vi "XVC_SERVER_UDP.vi"() -> ()   [LabVIEW 2017]
panel:
  out "error out":errorcluster
  in  "data out 5":string="shift:\u0005\u0000\u0000\u0000ÿ\u0000"
  out "received string 2":string
  in  "address":string="192.168.10.35"
  out "received string":string
  out "data out 3":string
  in  "data out 4":string="shift:\u0005\u0000\u0000\u0000ÿ\u0000"
  out "data out 2":string
  out "x != 0?":bool
  in  "Client Closed":string="The client VI closed the connection."
  in  "Stop":bool
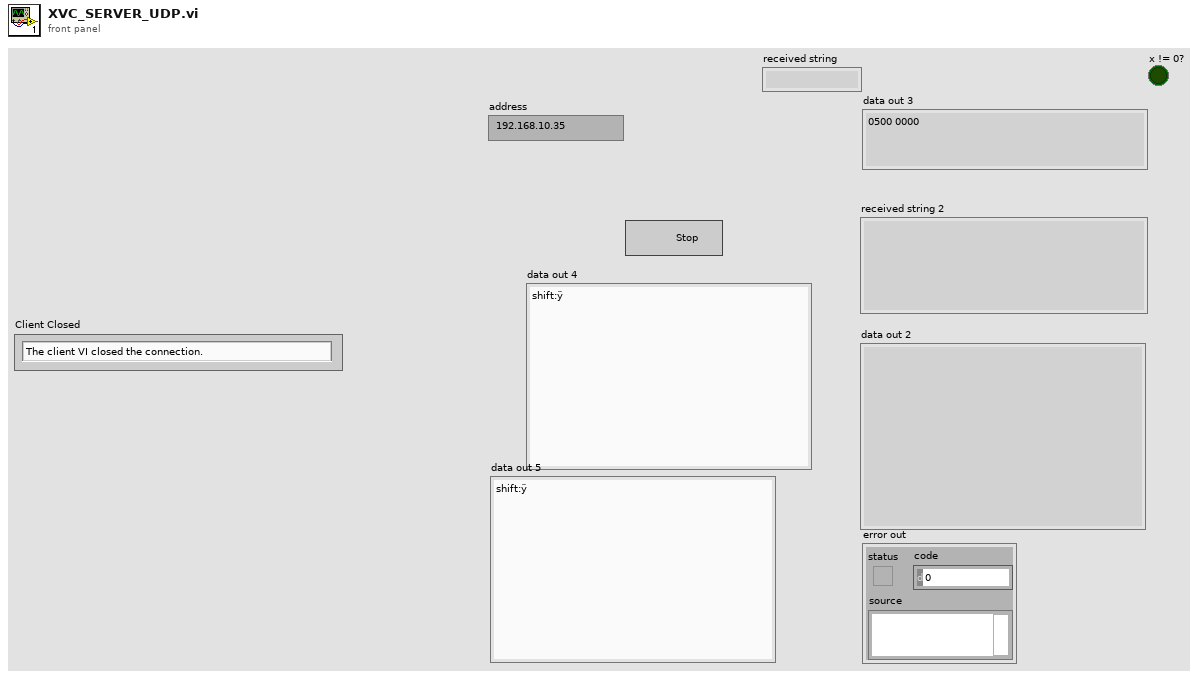
[diagram p1: front panel]
types:
  T1 = enum16{"Standard", "Buffered", "CRLF", "Immediate"}
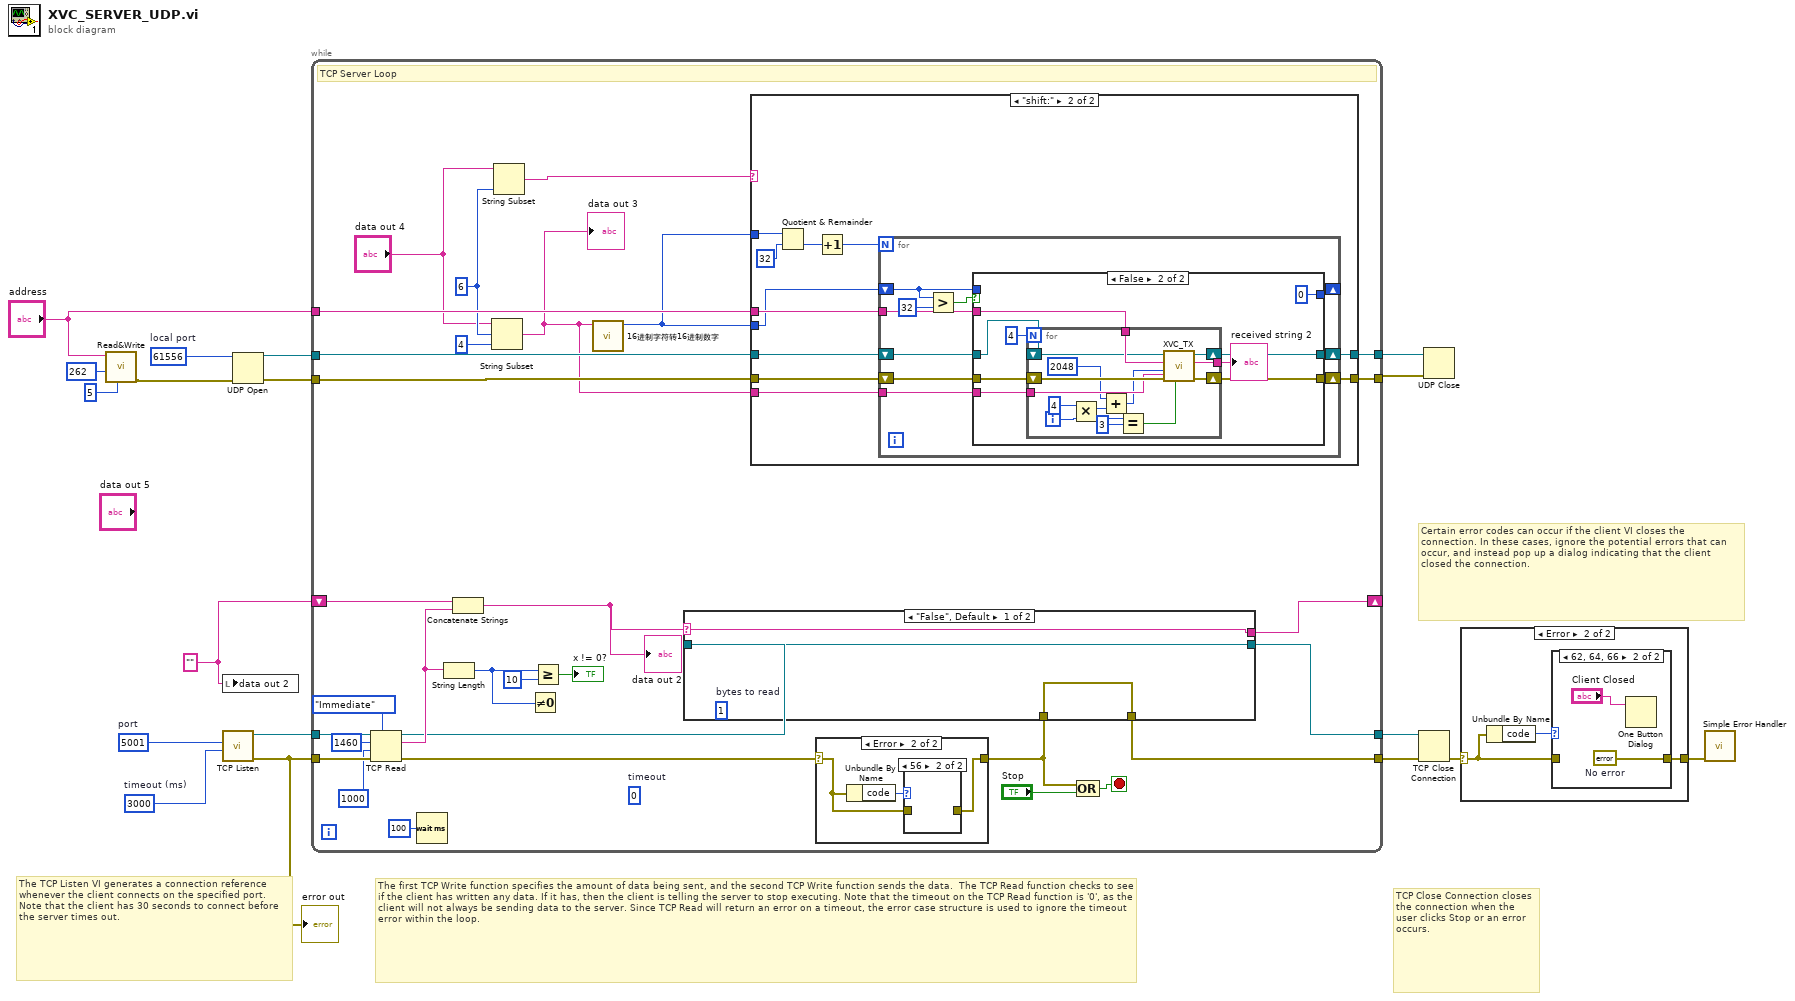
[diagram p0: block diagram]
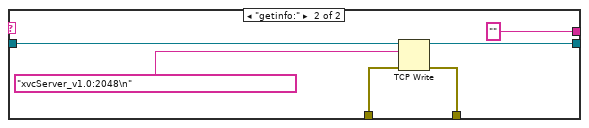
[diagram p4: hidden frame]
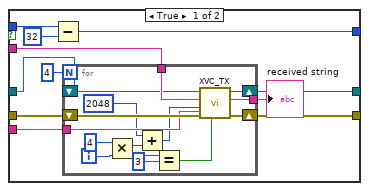
[diagram p6: hidden frame]
diagram:
  w10 = u16 61556  # local port
  w1 = ""
  w11 = u16 5001  # port
  w12 = 3000  # timeout (ms)
  # "TCP Close Connection closes the connection when the user clicks Stop or an error occurs."
  # "The TCP Listen VI generates a connection reference whenever the client connects on the specified port. Note that the client has 30 seconds to connect before the server times out."
  # "Certain error codes can occur if the client VI closes the connection. In these cases, ignore the potential errors that can occur, and instead pop up a dialog indicating that the client closed the connection."
  # "The first TCP Write function specifies the amount of data being sent, and the second TCP Write function sends the data.  The TCP Read function checks to see if the client has written any data. If it has, then the client is telling the server to stop executing. Note that the timeout on the TCP Read function is '0', as the client will not always be sending data to the server. Since TCP Read will return an error on a timeout, the error case structure is used to ignore the timeout error within the loop."
  n1 = call "Read&Write.vi"("In"=u8 5, "Address"=u32 262, "address"="address") -> ("error out"=w3:errorcluster)  [unwired: 7 in, 1 out]
  n2 = local write "data out 2"(w1) -> ()
  n3 = call <vilib>:"TCP Listen.vi"("timeout ms (wait forever: -1)"=w12, "port"=w11) -> ("error out"=w13:errorcluster, "connection ID"=w14:refnum<k5>)  [unwired: 5 in, 3 out]
  "error out" <- w13
  n4 = UDP Open(8:w3, 11:w10) -> (port=w9:refnum<k16>, 0:w8:errorcluster)  [unwired: 3 in, 1 out]
  n5 = while {
    tunnel: [w22] -> w17
    tunnel: [w20] -> w18
    tunnel: w14 -> [w49]
    tunnel: w13 -> [w46]
    shift-right: [w19] -> _
    shift-left: w1 -> [w41]
    tunnel: w9 -> [w35]
    tunnel: w8 -> [w29]
    tunnel: "address" -> [w37]
    tunnel: [w36] -> w7
    tunnel: [w33] -> w6
    stop <- w47 stop-if-true
    w30 = 6 ("length (rest)")
    (unwired) 0  # timeout
    (unwired) 1  # bytes to read
    # "TCP Server Loop"
    n6 = TCP Read(connection ID=w49, bytes to read=1460, error in (no error)=w46, 7:T1."Immediate" ("mode (standard)"), 9:1000 ("timeout ms (25000)")) -> (connection ID out=w21:refnum<k5>, data out=w40:string, error out=w44:errorcluster)
    n7 = Wait (ms)(milliseconds to wait=u32 100) -> ()  [unwired: 1 out]
    n8 = String Length(string=w40) -> (length=w38:i32)
    n9 = Concatenate Strings(w41, w40) -> (w24:string)
    "data out 2" <- w24
    n10 = String Subset(string="data out 4", offset (0)=w30, length (rest)=4 ("length (rest)")) -> (substring=w27:string)
    "data out 3" <- w27
    n11 = String Subset(string="data out 4", length (rest)=w30) -> (substring=w25:string)  [unwired: 1 in]
    n12 = Not Equal To 0?(x=w38) -> ()  [unwired: 1 out]
    n13 = Greater Or Equal?(x=w38, y=10) -> (x >= y?=→"x != 0?":bool)
    n14 = call "16进制字符转16进制数字.vi"("data in"=w27) -> ("number"=w26:u32)  [unwired: 10 in]
    n15 = case shown="\"shift:\"" w25 {
      tunnel: w37 -> [_ w71]
      tunnel: [w59 w69] -> w36
      tunnel: w35 -> [w60 w68]
      tunnel: [w60 w67] -> w33
      tunnel: w26 -> [_ w66]
      tunnel: w29 -> [w59 w70]
      tunnel: w27 -> [_ w62]
      tunnel: w26 -> [_ w61]
      frame "False", Default {
      }
      frame "shift:" {
        n16 = Quotient & Remainder(x=w66, y=u8 32) -> (floor(x/y)=w63:u32)  [unwired: 1 out]
        n17 = Increment(x=w63) -> (x+1=w64:u32)
        n18 = for {
          N: w64 -> [_]
          tunnel: w71 -> [w81]
          shift-right: [w79] -> w69
          shift-left: w70 -> [w80]
          shift-right: [w77] -> w67
          shift-left: w68 -> [w78]
          tunnel: w62 -> [w76]
          shift-right: [w72] -> _
          shift-left: w61 -> [w74]
          n19 = Greater?(x=w74, y=u32 32) -> (0:w75:bool)
          n20 = case shown="False" w75 {
            tunnel: w81 -> [w92 w115]
            tunnel: w80 -> [w91 w114]
            tunnel: [w90 w113] -> w79
            tunnel: w78 -> [w89 w112]
            tunnel: [w88 w111] -> w77
            tunnel: w76 -> [w87 w110]
            tunnel: w74 -> [w86 _]
            tunnel: [w84 u32 0] -> w72
            frame True {
              n21 = Subtract(x=w86, y=u32 32) -> (x-y=w84:u32)
              n22 = for {
                N: 4 -> [_]
                tunnel: w92 -> [w106]
                tunnel: w87 -> [w101]
                shift-right: [w104] -> w90
                shift-left: w91 -> [w105]
                shift-right: [w102] -> w88
                shift-left: w89 -> [w103]
                tunnel: [w93] -> w82
                i -> [w96]
                n23 = Multiply(x=4, y=w96) -> (x*y=w99:i32)
                n24 = Add(x=u32 2048 ("Address"), y=w99) -> (x+y=w97:u32)
                n25 = Equal?(x=w96, y=3) -> (x = y?=w94:bool)
                n26 = call "XVC_TX.vi"("data in"=w101, "Read (TRUE)"=w94, "error in"=w105, "Address"=w97, "IP address"=w106, "connection ID"=w103) -> ("error out"=w104:errorcluster, "received string"=w93:string, "connection ID 2"=w102:refnum<k16>)  [unwired: 3 in]
              }
              "received string" <- w82
            }
            frame False {
              n27 = for {
                N: 4 -> [_]
                tunnel: w115 -> [w129]
                tunnel: w110 -> [w124]
                shift-right: [w127] -> w113
                shift-left: w114 -> [w128]
                shift-right: [w125] -> w111
                shift-left: w112 -> [w126]
                tunnel: [w116] -> w108
                i -> [w119]
                n28 = Multiply(x=4, y=w119) -> (x*y=w122:i32)
                n29 = Add(x=u32 2048 ("Address"), y=w122) -> (x+y=w120:u32)
                n30 = Equal?(x=w119, y=3) -> (x = y?=w117:bool)
                n31 = call "XVC_TX.vi"("data in"=w124, "Read (TRUE)"=w117, "error in"=w128, "Address"=w120, "IP address"=w129, "connection ID"=w126) -> ("error out"=w127:errorcluster, "received string"=w116:string, "connection ID 2"=w125:refnum<k16>)  [unwired: 3 in]
              }
              "received string 2" <- w108
            }
          }
        }
      }
    }
    n32 = case shown="Error" w44 {
      selector: w44 -> [w130 w132]
      tunnel: [w130 w131] -> w23
      frame No Error {
      }
      frame Error {
        n33 = Unbundle By Name(w132) -> ("code"=w133:i32)
        n34 = case shown="56" w133 {
          tunnel: w132 -> [w134 _]
          tunnel: [w134 _] -> w131
          frame Default {
          }
          frame 56 {
          }
        }
      }
    }
    n35 = case shown="\"False\", Default" w24 {
      selector: w24 -> [w50 _]
      tunnel: w21 -> [w52 w58]
      tunnel: w23 -> [w51 w56]
      tunnel: [w51 w55] -> w22
      tunnel: [w52 w54] -> w20
      tunnel: [w50 ""] -> w19
      frame "False", Default {
      }
      frame "getinfo:" {
        n36 = TCP Write(connection ID=w58, data in="xvcServer_v1.0:2048\n", error in (no error)=w56) -> (connection ID out=w54:refnum<k5>, error out=w55:errorcluster)  [unwired: 1 in, 1 out]
      }
    }
    n37 = Compound Arithmetic op=OR(w23, "Stop") -> (w47:bool)
  }
  n38 = TCP Close Connection(connection ID=w18, error in (no error)=w17) -> (error out=w16:errorcluster)  [unwired: 2 out]
  n39 = UDP Close(connection ID=w6, 8:w7) -> ()  [unwired: 2 out]
  n40 = case shown="Error" w16 {
    selector: w16 -> [w135 w137]
    tunnel: [w135 w136] -> w15
    frame No Error {
    }
    frame Error {
      n41 = Unbundle By Name(w137) -> ("code"=w138:i32)
      n42 = case shown="62, 64, 66" w138 {
        tunnel: w137 -> [w139 _]
        tunnel: [w139 w141] -> w136
        frame Default {
        }
        frame 62, 64, 66 {
          w141 = errorcluster {"status"=FALSE, "code"=0, "source"=""}  # No error
          n43 = One Button Dialog(message="Client Closed") -> ()  [unwired: 1 in, 1 out]
        }
      }
    }
  }
  n44 = call <vilib>:"Simple Error Handler.vi"("error in (no error)"=w15) -> ()  [unwired: 1 in, 8 out]
